vi "PatientGlobals.vi"() -> ()   [LabVIEW 2022 SP3]
uses:
  Real Time/-RT_support/PatientInfoDef.ctl
  LymphNodeInfo.ctl
  TissueTypeScan.ctl
panel:
  in  "Node Info":T1 {"Year" format="%02d"; "Patient Number" format="%03d"; "Node Number" format="%02d"}
  in  "Patient ID":string="temp"
  in  "Patient Info":T3={"Eye Selector"=enum."Right", "Plane"=1, "First Name"="", "Last Name"="", "Notes"="", "Patient ID"="", "Scan Location"=enum."Radio Selection 1"} {"Plane" min=1 max=12 step=1 scale=0.0..12.0}
  in  "Database Path":path=path "D:/Temp"
  out "PatientFileName":string
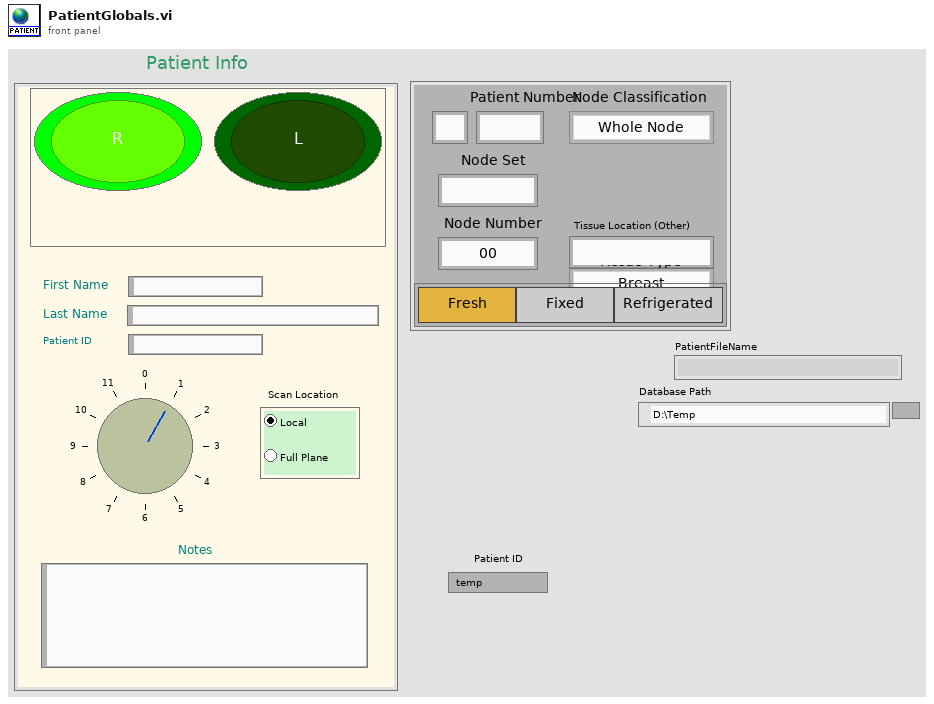
[diagram p1: front panel]
types:
  T1 = typedef "LymphNodeInfo.ctl" = cluster{"Patient Number":u32, "Node Set":string, "Node Number":u32, "Tissue Type":T2, "Tissue Location (Other)":string, "Node Classification":enum16{"Whole Node", "Piece A", "Piece B", "Piece C"}, "Fresh?":enum32{"Fresh?", "Fixed?", "Refrigerated?"}, "Year":u32}
  T2 = typedef "TissueTypeScan.ctl" = enum16{"Breast", "Gastric", "Stomach", "Rectal", "Colon", "Head & Neck", "Other"}
  T3 = typedef "PatientInfoDef.ctl" = cluster{"Eye Selector":enum32{"Left", "Right"}, "Plane":i8, "First Name":string, "Last Name":string, "Notes":string, "Patient ID":string, "Scan Location":enum32{"Radio Selection 1", "Radio Selection 2"}}
diagram:
